vi "fetch_and_translate_trigger.vi"(8 "error in (no error)":errorcluster, 11 "DataCollectionDL091104Scaffold in":refnum<class "DataCollectionDL091104Scaffold.lvclass">) -> (0 "error out":errorcluster, 1 "sender TLC type":T1, 2 "trigger":T2=enum."initialise", 3 "DataCollectionDL091104Scaffold out":refnum<class "DataCollectionDL091104Scaffold.lvclass">)   [LabVIEW 2010, in "DataCollectionDL091104Scaffold.lvclass"]
uses:
  DataCollectionDL091104Scaffold.lvclass
  action_enum.ctl
  common/enumerations/top-level_component_type_enum.ctl
  GenericDataCollection/GenericDataCollection/trigger_enum.ctl
  GenericDataCollection/GenericDataCollection/GenericDataCollection.lvclass
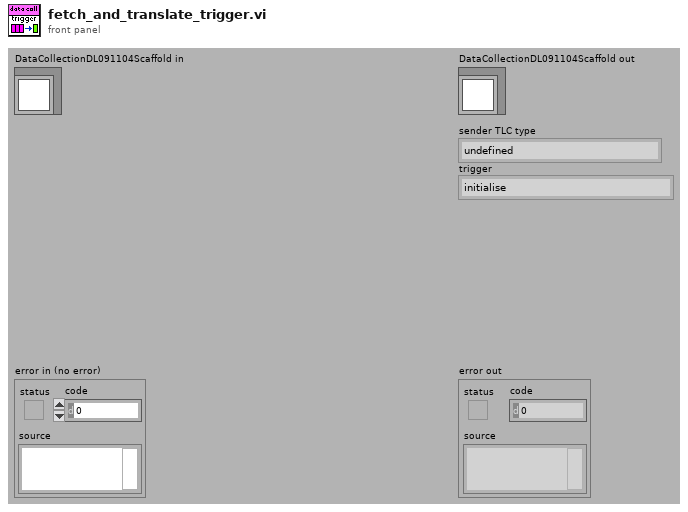
[diagram p1: front panel]
types:
  T1 = typedef "top-level_component_type_enum.ctl" = enum16{"undefined", "ImagingMode", "ScanHead", "DAQ", "ImageAssembler", "Display", "DataCollection", "Analyser", "Stimulator", "ExperimentController", "Instrument", "Stage"}
  T2 = typedef "DataCollectionDL091104Scaffold.lvclass/action_enum.ctl" = enum16{"NULL", "initialise", "terminate", "reset", "insert", "save", "register as observer", "sweep finished", "attach observer", "detach observer"}
  T3 = typedef "GenericDataCollection.lvclass/trigger_enum.ctl" = enum16{"NULL", "save", "reset"}
  T4 = typedef "GenericToplevelComponent.lvclass/common_trigger_enum.ctl" = enum16{"NULL", "initialise", "terminate", "fetch command", "fetch data", "attach observer", "register as observer", "detach observer", "acknowledge", "start", "stop", "sweep started", "sweep finished", "experiment started", "experiment stopped"}
  T5 = typedef "trigger_type_enum.ctl" = enum8{"external", "internal", "common"}
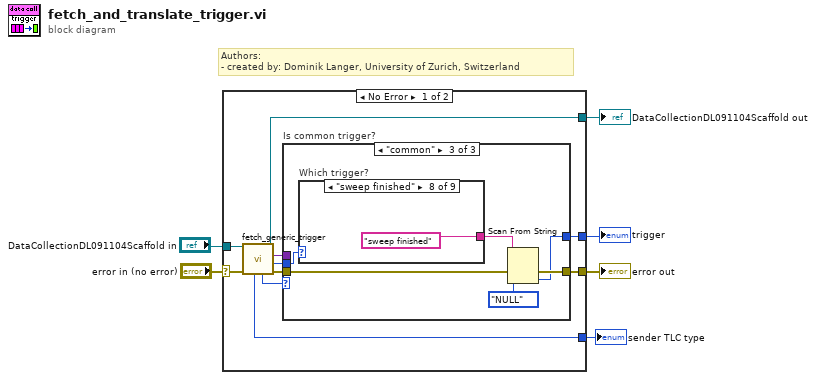
[diagram p0: block diagram]
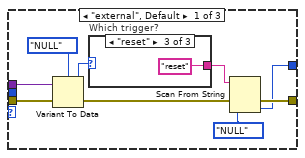
[diagram p2: hidden frame]
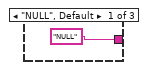
[diagram p3: hidden frame]
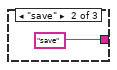
[diagram p4: hidden frame]
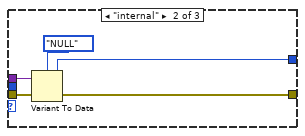
[diagram p5: hidden frame]
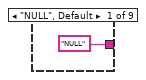
[diagram p6: hidden frame]
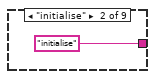
[diagram p7: hidden frame]
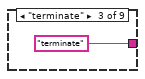
[diagram p8: hidden frame]
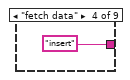
[diagram p9: hidden frame]
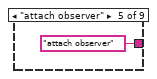
[diagram p10: hidden frame]
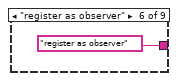
[diagram p11: hidden frame]
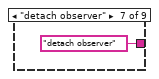
[diagram p12: hidden frame]
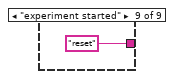
[diagram p13: hidden frame]
diagram:
  # "Authors: \n- created by: Dominik Langer, University of Zurich, Switzerland"
  n1 = case shown="No Error" "error in (no error)" {
    selector: "error in (no error)" -> [w14 w50]
    tunnel: [w16 w50] -> w5
    tunnel: [w11 w49] -> w3
    tunnel: "DataCollectionDL091104Scaffold in" -> [w12 w49]
    tunnel: [w15 _] -> w1
    tunnel: [w7 _] -> w2
    frame No Error {
      n2 = call-dynamic "fetch_generic_trigger.vi"("error in (no error)"=w14, "GenericToplevelComponent in"=w12) -> ("error out"=w13:errorcluster, "common trigger"=w8:T4, "trigger"=w10:variant, "GenericToplevelComponent out"=w11:refnum<class "DataCollectionDL091104Scaffold.lvclass">, "trigger type"=w9:T5, "sender TLC type"=w7:T1)  [unwired: 3 in, 1 out]
      n3 = case "Is common trigger?" shown="\"common\"" w9 {
        tunnel: [w19 w32 w36] -> w16
        tunnel: [w17 w30 w34] -> w15
        tunnel: w13 -> [w23 w33 w38]
        tunnel: w10 -> [w22 w31 _]
        tunnel: w8 -> [_ _ w39]
        frame "external", Default {
          n4 = Variant To Data(error in=w23, Variant=w22, type=trigger_enum."NULL" ("trigger")) -> (error out=w20:errorcluster, data=w24:T3)
          n5 = case "Which trigger?" shown="\"reset\"" w24 {
            tunnel: ["NULL" "save" "reset"] -> w21
            frame "NULL", Default {
            }
            frame "save" {
            }
            frame "reset" {
            }
          }
          n6 = Scan From String(input string=w21, error in=w20, default 1=action_enum."NULL" ("trigger")) -> (error out=w19:errorcluster, output 1=w17:T2)  [unwired: 2 in, 2 out]
        }
        frame "internal" {
          n7 = Variant To Data(error in=w33, Variant=w31, type=action_enum."NULL" ("trigger")) -> (error out=w32:errorcluster, data=w30:T2)
        }
        frame "common" {
          n8 = case "Which trigger?" shown="\"sweep finished\"" w39 {
            tunnel: ["NULL" "initialise" "terminate" "insert" "attach observer" "register as observer" "detach observer" "sweep finished" "reset"] -> w37
            frame "NULL", Default {
            }
            frame "initialise" {
            }
            frame "terminate" {
            }
            frame "fetch data" {
            }
            frame "attach observer" {
            }
            frame "register as observer" {
            }
            frame "detach observer" {
            }
            frame "sweep finished" {
            }
            frame "experiment started" {
            }
          }
          n9 = Scan From String(input string=w37, error in=w38, default 1=action_enum."NULL" ("trigger")) -> (error out=w36:errorcluster, output 1=w34:T2)  [unwired: 2 in, 2 out]
        }
      }
    }
    frame Error {
    }
  }
  "error out" <- w5
  "DataCollectionDL091104Scaffold out" <- w3
  "trigger" <- w1
  "sender TLC type" <- w2
